vi "ADCP_Close_Node_Connection.vi"(8 "error in (no error)":errorcluster, 10 "Node ID":i32=-1, 11 "ADCP In":refnum<class "ADCP.lvclass">) -> (0 "error out":errorcluster, 3 "ADCP Out":refnum<class "ADCP.lvclass">)   [LabVIEW 2017, in "ADCP.lvclass"]
uses:
  ADCP.lvclass
  ADCP.lvclass/ADCP.ctl
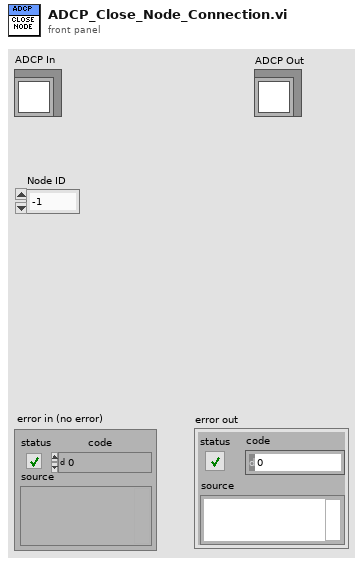
[diagram p1: front panel]
types:
  T1 = cluster{"CC_ACK":bool, "CC_RQST":bool, "OC_ACK":bool, "OC_RQST":bool, "SYNC_ACK":bool, "SYNC_RQST":bool}
  T2 = enum16{"NONE", "CONNECTION_ALREADY_OPEN", "CONNECTION_ALREADY_CLOSED", "INVALID_FRAME_REQUEST"}
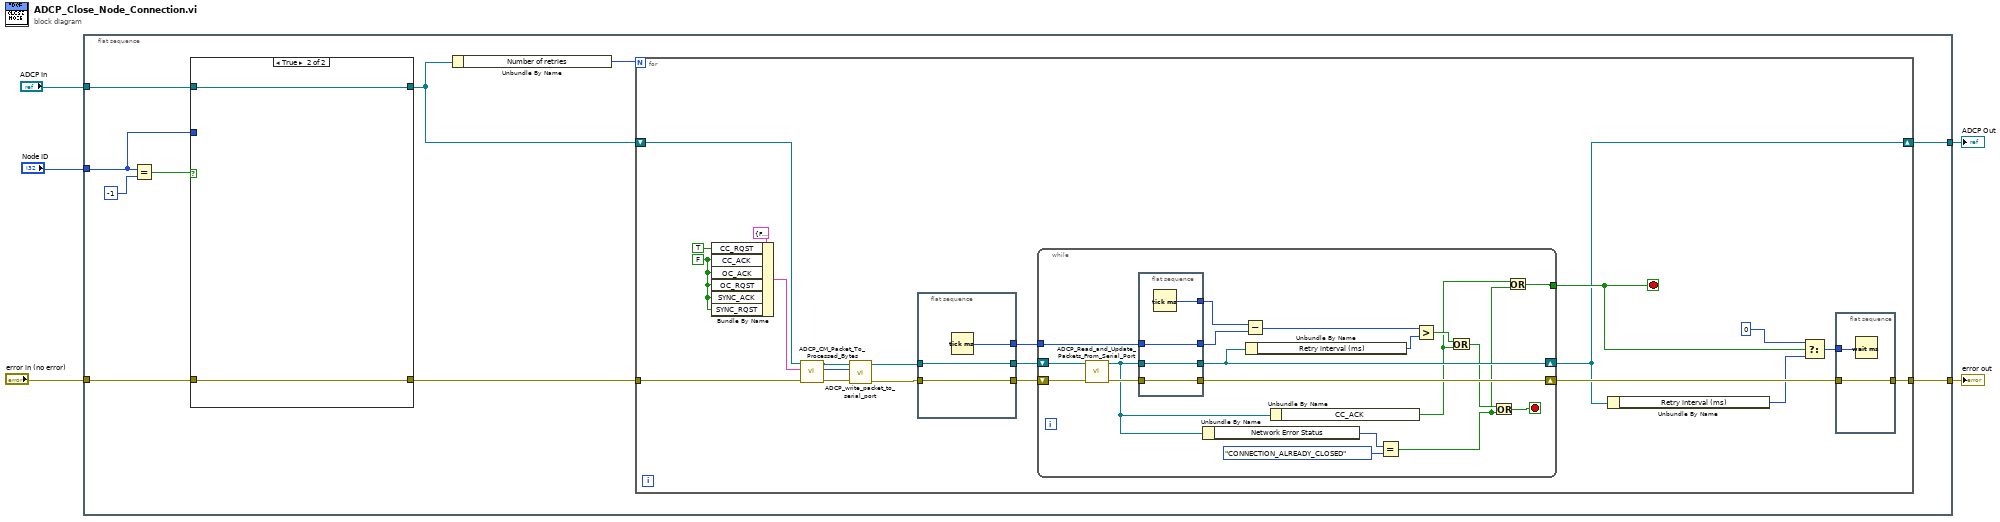
[diagram p0: block diagram]
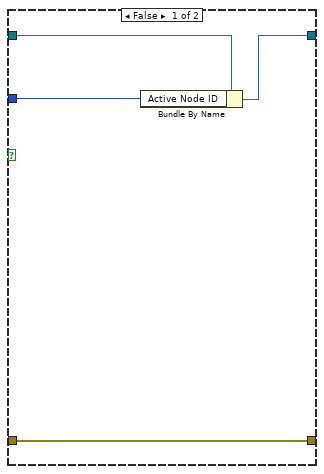
[diagram p2: hidden frame]
diagram:
  n1 = flat-sequence {
    tunnel: "ADCP In" -> [w12]
    tunnel: "error in (no error)" -> [w14]
    tunnel: "Node ID" -> [w11]
    tunnel: [w7] -> w2
    tunnel: [w6] -> w1
    frame #0 {
      n2 = Equal?(x=w11, y=-1) -> (x = y?=w13:bool)
      n3 = case shown="True" w13 {
        tunnel: w14 -> [w65 w69]
        tunnel: w12 -> [w68 w70]
        tunnel: [w66 w70] -> w8
        tunnel: w11 -> [w67 _]
        tunnel: [w65 w69] -> w10
        frame False {
          n4 = Bundle By Name(cluster=w68, "Active Node ID"=w67) -> (w66:refnum<class "ADCP.lvclass">)
        }
        frame True {
        }
      }
      n5 = Unbundle By Name(w8) -> ("Number of retries"=w9:u16)
      n6 = for {
        N: w9 -> [_]
        tunnel: w10 -> [w36]
        shift-right: [w23] -> w7
        shift-left: w8 -> [w35]
        tunnel: [w21] -> w6
        stop <- w26 stop-if-true
        w31 = FALSE ("OC_ACK")
        n7 = Bundle By Name(cluster=T1 {"CC_ACK"=FALSE, "CC_RQST"=FALSE, "OC_ACK"=FALSE, "OC_RQST"=FALSE, "SYNC_ACK"=FALSE, "SYNC_RQST"=FALSE} ("ADCP Connection Management Packet"), "CC_RQST"=TRUE ("OC_ACK"), "CC_ACK"=w31, "OC_ACK"=w31, "OC_RQST"=w31, "SYNC_ACK"=w31, "SYNC_RQST"=w31) -> (w32:T1)
        n8 = call "ADCP_CM_Packet_To_Processed_Bytes.vi"("error in (no error)"=w36, "Connection Management"=w32, "ADCP in"=w35) -> ("error out"=w18:errorcluster, "Processed Packet"=w20:u8[], "ADCP out"=w19:refnum<class "ADCP.lvclass">)  [unwired: 6 in]
        n9 = call "ADCP_write_packet_to_serial_port.vi"("error in (no error)"=w18, "Packet Bytes"=w20, "ADCP In"=w19) -> ("error out"=w17:errorcluster, "ADCP Out"=w16:refnum<class "ADCP.lvclass">)  [unwired: 7 in]
        n10 = flat-sequence {
          tunnel: w16 -> [w41]
          tunnel: [w41] -> w30
          tunnel: w17 -> [w40]
          tunnel: [w40] -> w29
          tunnel: [w39] -> w28
          frame #0 {
            n11 = Tick Count (ms)() -> (millisecond timer value=w39:u32)
          }
        }
        n12 = while {
          shift-right: [w52] -> w23
          shift-left: w30 -> [w59]
          shift-right: [w57] -> w27
          shift-left: w29 -> [w60]
          tunnel: w28 -> [w55]
          tunnel: [w42] -> w26
          stop <- w45 stop-if-true
          n13 = call "ADCP_Read_and_Update_Packets_From_Serial_Port.vi"("error in (no error)"=w60, "ADCP In"=w59) -> ("error out"=w58:errorcluster, "ADCP out"=w49:refnum<class "ADCP.lvclass">)  [unwired: 6 in, 2 out]
          n14 = flat-sequence {
            tunnel: w49 -> [w64]
            tunnel: [w64] -> w52
            tunnel: w58 -> [w63]
            tunnel: [w63] -> w57
            tunnel: [w62] -> w56
            tunnel: w55 -> [w61]
            tunnel: [w61] -> w54
            frame #0 {
              n15 = Tick Count (ms)() -> (millisecond timer value=w62:u32)
            }
          }
          n16 = Unbundle By Name(w49) -> ("Network Error Status"=w48:T2)
          n17 = Subtract(x=w56, y=w54) -> (x-y=w53:u32)
          n18 = Unbundle By Name(w52) -> ("Retry interval (ms)"=w51:u16)
          n19 = Unbundle By Name(w49) -> ("CC_ACK"=w44:bool)
          n20 = Equal?(x=w48, y=T2."CONNECTION_ALREADY_CLOSED") -> (x = y?=w43:bool)
          n21 = Greater?(x=w53, y=w51) -> (0:w50:bool)
          n22 = Or(x=w50, y=w44) -> (x .or. y?=w46:bool)
          n23 = Or(x=w46, y=w43) -> (x .or. y?=w45:bool)
          n24 = Or(x=w44, y=w43) -> (x .or. y?=w42:bool)
        }
        n25 = Unbundle By Name(w23) -> ("Retry interval (ms)"=w22:u16)
        n26 = Select(t=0, s=w26, f=w22) -> (s? t:f=w24:i32)
        n27 = flat-sequence {
          tunnel: w27 -> [w38]
          tunnel: [w38] -> w21
          tunnel: w24 -> [w37]
          frame #0 {
            n28 = Wait (ms)(milliseconds to wait=w37) -> ()  [unwired: 1 out]
          }
        }
      }
    }
  }
  "ADCP Out" <- w2
  "error out" <- w1
